vi "Cleanup With Fade Out.vi"(8 "error in (no error)":errorcluster, 11 "Flex Dialog in":refnum<class "Flex UI Dialog.lvclass">) -> (0 "error out":errorcluster, 3 "Flex Dialog out":refnum<class "Flex UI Dialog.lvclass">)   [LabVIEW 2016, in "Flex UI Dialog.lvclass"]
uses:
  Flex UI Dialog.lvclass
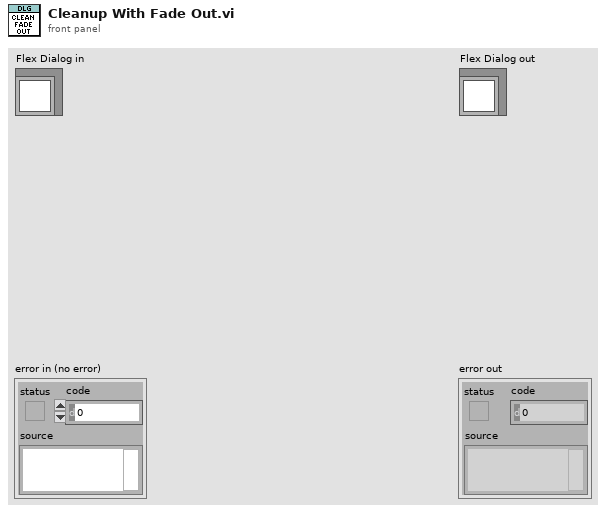
[diagram p1: front panel]
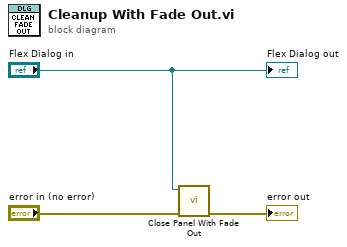
[diagram p0: block diagram]
diagram:
  n1 = call-dynamic "Close Panel With Fade Out.vi"("error in"="error in (no error)", "Flex Dialog in"="Flex Dialog in") -> ("error out"=→"error out":errorcluster)  [unwired: 8 in, 1 out]
  "Flex Dialog out" <- "Flex Dialog in"
